vi "RPC Version.vi"(8 "error in (no error)":errorcluster, 11 "Identified in":refnum<class "Identified.lvclass">) -> (0 "error out":errorcluster, 2 "RPC Version":i32, 3 "Identified out":refnum<class "Identified.lvclass">)   [LabVIEW 2020, in "obs-websocket.lvlib" / "Identified.lvclass"]
uses:
  Identified.lvclass
  Identified.lvclass/Identified.ctl
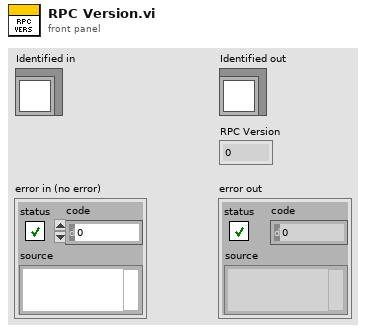
[diagram p1: front panel]
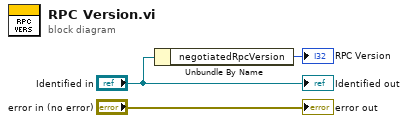
[diagram p0: block diagram]
diagram:
  n1 = Unbundle By Name("Identified in") -> ("negotiatedRpcVersion"=→"RPC Version":i32)
  "error out" <- "error in (no error)"
  "Identified out" <- "Identified in"
